vi "iRobot Read Sensor Group 6.vi"(11 "stream in":u8[](array[numeric])) -> (1 "iRobot Sensor Group 6":T1 {"Infrared" format="%02x"}, 3 "stream out":u8[](array[numeric]))   [LabVIEW 2010]
doc: "Read Sensor Group 6 from a UART data stream."
uses:
  Sensor Controls/iRobot Sensor Group 6.ctl
  Sensor Controls/iRobot Bumps + Wheel Drops.ctl
  Sensor Controls/iRobot Low-Side Driver + Wheel Overcurrent.ctl
  Sensor Controls/iRobot Buttons.ctl
  Sensor Controls/iRobot Charging State.ctl
  Sensor Controls/iRobot Cargo Bay Digital Inputs.ctl
  Sensor Controls/iRobot Charging Sources Available.ctl
  Sensor Controls/iRobot OI Mode.ctl
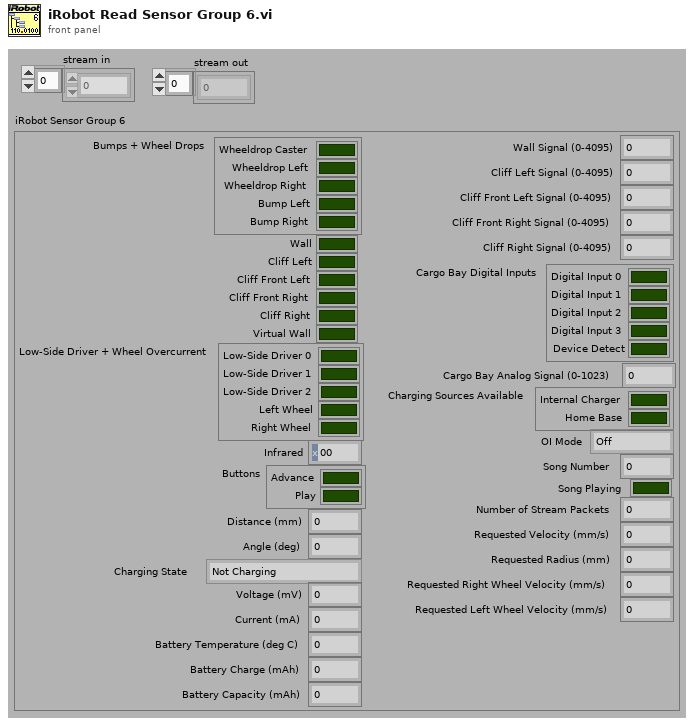
[diagram p1: front panel]
types:
  T1 = typedef "iRobot Sensor Group 6.ctl" = cluster{"Bumps + Wheel Drops":T2, "Wall":bool, "Cliff Left":bool, "Cliff Front Left":bool, "Cliff Front Right":bool, "Cliff Right":bool, "Virtual Wall":bool, "Low-Side Driver + Wheel Overcurrent":T3, "Infrared":u8, "Buttons":T4, "Distance (mm)":i32, "Angle (deg)":i32, "Charging State":T5, "Voltage (mV)":u16, "Current (mA)":i16, "Battery Temperature (deg C)":i8, "Battery Charge (mAh)":u16, "Battery Capacity (mAh)":u16, "Wall Signal (0-4095)":u16, "Cliff Left Signal (0-4095)":u16, "Cliff Front Left Signal (0-4095)":u16, "Cliff Front Right Signal (0-4095)":u16, "Cliff Right Signal (0-4095)":u16, "Cargo Bay Digital Inputs":T6, "Cargo Bay Analog Signal (0-1023)":u16, "Charging Sources Available":T7, "OI Mode":T8, "Song Number":u8, "Song Playing":bool, "Number of Stream Packets":u8, "Requested Velocity (mm/s)":u8, "Requested Radius (mm)":u8, "Requested Right Wheel Velocity (mm/s)":u8, "Requested Left Wheel Velocity (mm/s)":u8}
  T2 = typedef "iRobot Bumps + Wheel Drops.ctl" = cluster{"Wheeldrop Caster":bool, "Wheeldrop Left":bool, "Wheeldrop Right":bool, "Bump Left":bool, "Bump Right":bool}
  T3 = typedef "iRobot Low-Side Driver + Wheel Overcurrent.ctl" = cluster{"Low-Side Driver 0":bool, "Low-Side Driver 1":bool, "Low-Side Driver 2":bool, "Left Wheel":bool, "Right Wheel":bool}
  T4 = typedef "iRobot Buttons.ctl" = cluster{"Advance":bool, "Play":bool}
  T5 = typedef "iRobot Charging State.ctl" = enum16{"Not Charging", "Reconditioning Charging", "Full Charging", "Trickle Charging", "Waiting", "Charging Fault Condition"}
  T6 = typedef "iRobot Cargo Bay Digital Inputs.ctl" = cluster{"Digital Input 0":bool, "Digital Input 1":bool, "Digital Input 2":bool, "Digital Input 3":bool, "Device Detect":bool}
  T7 = typedef "iRobot Charging Sources Available.ctl" = cluster{"Internal Charger":bool, "Home Base":bool}
  T8 = typedef "iRobot OI Mode.ctl" = enum16{"Off", "Passive", "Safe", "Full"}
  T9 = typedef "iRobot Sensor Group 0.ctl" = cluster{"Bumps + Wheel Drops":T2, "Wall":bool, "Cliff Left":bool, "Cliff Front Left":bool, "Cliff Front Right":bool, "Cliff Right":bool, "Virtual Wall":bool, "Low-Side Driver + Wheel Overcurrent":T3, "Infrared":u8, "Buttons":T4, "Distance (mm)":i32, "Angle (deg)":i32, "Charging State":T5, "Voltage (mV)":u16, "Current (mA)":i16, "Battery Temperature (deg C)":i8, "Battery Charge (mAh)":u16, "Battery Capacity (mAh)":u16}
  T10 = typedef "iRobot Sensor Group 4.ctl" = cluster{"Wall Signal (0-4095)":u16, "Cliff Left Signal (0-4095)":u16, "Cliff Front Left Signal (0-4095)":u16, "Cliff Front Right Signal (0-4095)":u16, "Cliff Right Signal (0-4095)":u16, "Cargo Bay Digital Inputs":T6, "Cargo Bay Analog Signal (0-1023)":u16, "Charging Sources Available":T7}
  T11 = typedef "iRobot Sensor Group 5.ctl" = cluster{"OI Mode":T8, "Song Number":u8, "Song Playing":bool, "Number of Stream Packets":u8, "Requested Velocity (mm/s)":u8, "Requested Radius (mm)":u8, "Requested Right Wheel Velocity (mm/s)":u8, "Requested Left Wheel Velocity (mm/s)":u8}
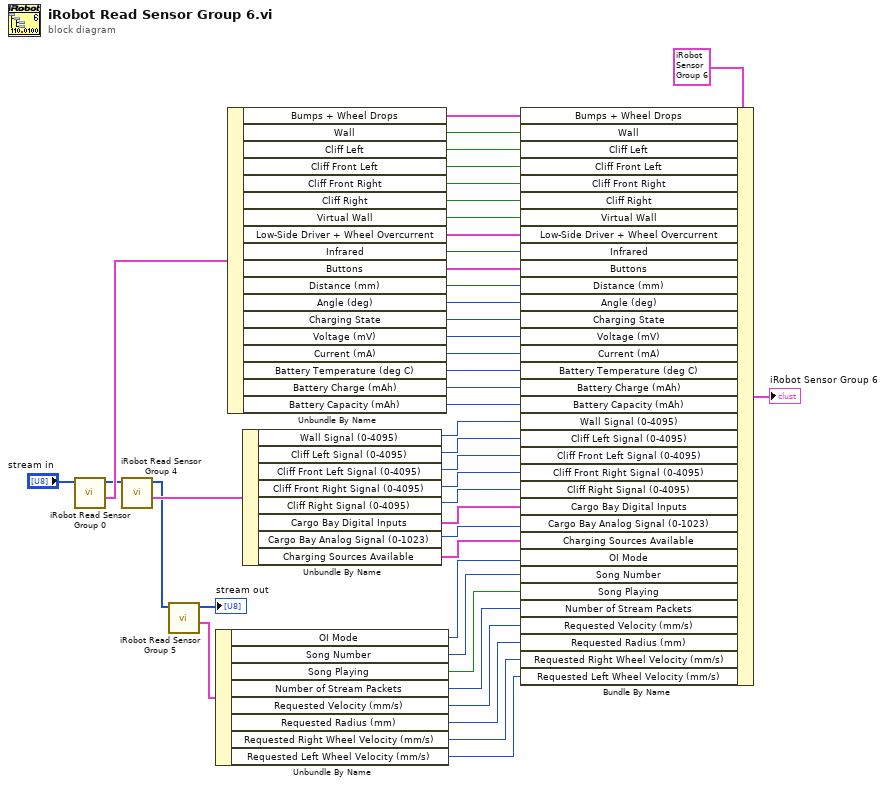
[diagram p0: block diagram]
diagram:
  n1 = call "iRobot Read Sensor Group 0.vi"("stream in"="stream in") -> ("Sensor Group 0"=w41:T9, "stream out"=w22:u8[])  [unwired: 9 out]
  n2 = call "iRobot Read Sensor Group 4.vi"("stream in"=w22) -> ("Sensor Group 4"=w21:T10, "stream out"=w15:u8[])  [unwired: 9 out]
  n3 = call "iRobot Read Sensor Group 5.vi"("stream in"=w15) -> ("Sensor Group 5"=w13:T11, "stream out"=→"stream out":u8[])  [unwired: 9 out]
  n4 = Unbundle By Name(w13) -> ("OI Mode"=w9:T8, "Song Number"=w8:u8, "Song Playing"=w7:bool, "Number of Stream Packets"=w6:u8, "Requested Velocity (mm/s)"=w5:u8, "Requested Radius (mm)"=w4:u8, "Requested Right Wheel Velocity (mm/s)"=w3:u8, "Requested Left Wheel Velocity (mm/s)"=w2:u8)
  n5 = Unbundle By Name(w41) -> ("Bumps + Wheel Drops"=w40:T2, "Wall"=w39:bool, "Cliff Left"=w38:bool, "Cliff Front Left"=w37:bool, "Cliff Front Right"=w36:bool, "Cliff Right"=w35:bool, "Virtual Wall"=w34:bool, "Low-Side Driver + Wheel Overcurrent"=w33:T3, "Infrared"=w32:u8, "Buttons"=w31:T4, "Distance (mm)"=w30:i32, "Angle (deg)"=w29:i32, "Charging State"=w28:T5, "Voltage (mV)"=w27:u16, "Current (mA)"=w26:i16, "Battery Temperature (deg C)"=w25:i8, "Battery Charge (mAh)"=w24:u16, "Battery Capacity (mAh)"=w23:u16)
  n6 = Unbundle By Name(w21) -> ("Wall Signal (0-4095)"=w20:u16, "Cliff Left Signal (0-4095)"=w19:u16, "Cliff Front Left Signal (0-4095)"=w18:u16, "Cliff Front Right Signal (0-4095)"=w17:u16, "Cliff Right Signal (0-4095)"=w16:u16, "Cargo Bay Digital Inputs"=w12:T6, "Cargo Bay Analog Signal (0-1023)"=w11:u16, "Charging Sources Available"=w10:T7)
  n7 = Bundle By Name(cluster=T1 {"Bumps + Wheel Drops"={"Wheeldrop Caster"=FALSE, "Wheeldrop Left"=FALSE, "Wheeldrop Right"=FALSE, "Bump Left"=FALSE, "Bump Right"=FALSE}, "Wall"=FALSE, "Cliff Left"=FALSE, "Cliff Front Left"=FALSE, "Cliff Front Right"=FALSE, "Cliff Right"=FALSE, "Virtual Wall"=FALSE, "Low-Side Driver + Wheel Overcurrent"={"Low-Side Driver 0"=FALSE, "Low-Side Driver 1"=FALSE, "Low-Side Driver 2"=FALSE, "Left Wheel"=FALSE, "Right Wheel"=FALSE}, "Infrared"=0, "Buttons"={"Advance"=FALSE, "Play"=FALSE}, "Distance (mm)"=0, "Angle (deg)"=0, "Charging State"=enum."Not Charging", "Voltage (mV)"=0, "Current (mA)"=0, "Battery Temperature (deg C)"=0, "Battery Charge (mAh)"=0, "Battery Capacity (mAh)"=0, "Wall Signal (0-4095)"=0, "Cliff Left Signal (0-4095)"=0, "Cliff Front Left Signal (0-4095)"=0, "Cliff Front Right Signal (0-4095)"=0, "Cliff Right Signal (0-4095)"=0, "Cargo Bay Digital Inputs"={"Digital Input 0"=FALSE, "Digital Input 1"=FALSE, "Digital Input 2"=FALSE, "Digital Input 3"=FALSE, "Device Detect"=FALSE}, "Cargo Bay Analog Signal (0-1023)"=0, "Charging Sources Available"={"Internal Charger"=FALSE, "Home Base"=FALSE}, "OI Mode"=enum."Off", "Song Number"=0, "Song Playing"=FALSE, "Number of Stream Packets"=0, "Requested Velocity (mm/s)"=0, "Requested Radius (mm)"=0, "Requested Right Wheel Velocity (mm/s)"=0, "Requested Left Wheel Velocity (mm/s)"=0} ("iRobot Sensor Group 6"), "Bumps + Wheel Drops"=w40, "Wall"=w39, "Cliff Left"=w38, "Cliff Front Left"=w37, "Cliff Front Right"=w36, "Cliff Right"=w35, "Virtual Wall"=w34, "Low-Side Driver + Wheel Overcurrent"=w33, "Infrared"=w32, "Buttons"=w31, "Distance (mm)"=w30, "Angle (deg)"=w29, "Charging State"=w28, "Voltage (mV)"=w27, "Current (mA)"=w26, "Battery Temperature (deg C)"=w25, "Battery Charge (mAh)"=w24, "Battery Capacity (mAh)"=w23, "Wall Signal (0-4095)"=w20, "Cliff Left Signal (0-4095)"=w19, "Cliff Front Left Signal (0-4095)"=w18, "Cliff Front Right Signal (0-4095)"=w17, "Cliff Right Signal (0-4095)"=w16, "Cargo Bay Digital Inputs"=w12, "Cargo Bay Analog Signal (0-1023)"=w11, "Charging Sources Available"=w10, "OI Mode"=w9, "Song Number"=w8, "Song Playing"=w7, "Number of Stream Packets"=w6, "Requested Velocity (mm/s)"=w5, "Requested Radius (mm)"=w4, "Requested Right Wheel Velocity (mm/s)"=w3, "Requested Left Wheel Velocity (mm/s)"=w2) -> (→"iRobot Sensor Group 6":T1)
